vi "GaGeError.vi"(6 "Ingnore no sytem":bool=TRUE, 7 "source":string, 8 "error in (no error)":errorcluster, 9 "StopOnError (false)":bool, 10 "Error Code":i32, 11 "Handle Cluster":T1) -> (0 "error out":errorcluster, 3 "Error String":string)   [LabVIEW 2015]
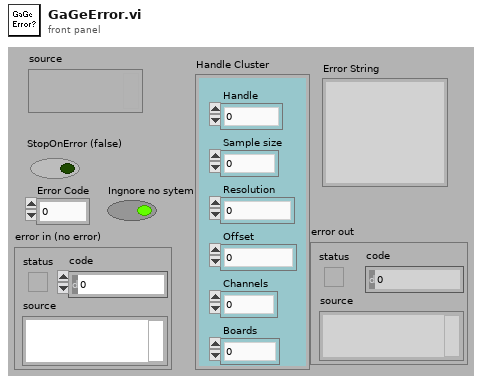
[diagram p1: front panel]
types:
  T1 = cluster{"Handle":u32, "Sample size":u32, "Resolution":i32, "Offset":i32, "Channels":u32, "Boards":u32}
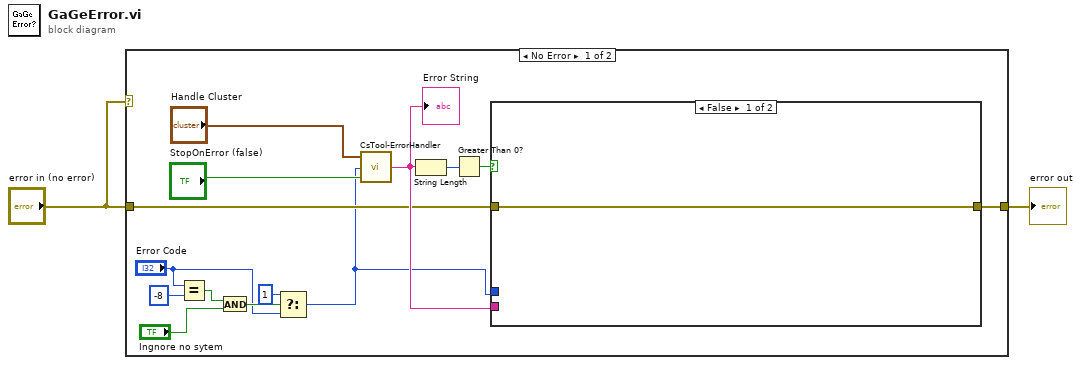
[diagram p0: block diagram]
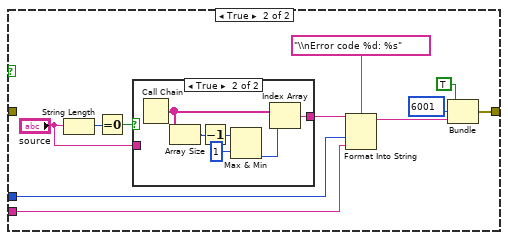
[diagram p2: hidden frame]
diagram:
  n1 = case shown="No Error" "error in (no error)" {
    tunnel: "error in (no error)" -> [w11 w36]
    tunnel: [w10 w36] -> w1
    frame No Error {
      n2 = Equal?(x="Error Code", y=-8) -> (x = y?=w8:bool)
      n3 = And(x=w8, y="Ingnore no sytem") -> (x .and. y?=w6:bool)
      n4 = Select(t=1, s=w6, f="Error Code") -> (s? t:f=w3:i32)
      n5 = call "CsTool-ErrorHandler.vi"("StopOnError (true)"="StopOnError (false)", "Error Code"=w3, "Handle Cluster"="Handle Cluster") -> ("Error String"=w12:string)
      "Error String" <- w12
      n6 = String Length(string=w12) -> (length=w14:i32)
      n7 = Greater Than 0?(x=w14) -> (x > 0?=w13:bool)
      n8 = case shown="False" w13 {
        tunnel: w3 -> [_ w20]
        tunnel: w12 -> [_ w19]
        tunnel: w11 -> [w17 _]
        tunnel: [w17 w18] -> w10
        frame False {
        }
        frame True {
          n9 = String Length(string="source") -> (length=w26:i32)
          n10 = Equal To 0?(x=w26) -> (x = 0?=w25:bool)
          n11 = case shown="True" w25 {
            tunnel: [w29 w33] -> w23
            tunnel: "source" -> [w29 _]
            frame False {
            }
            frame True {
              n12 = Call Chain() -> (call chain=w34:string[])
              n13 = Array Size(array=w34) -> (size(s)=w35:i32)
              n14 = Decrement(x=w35) -> (x-1=w32:i32)
              n15 = Max & Min(x=w32, y=1) -> (min(x,y)=w31:i32)  [unwired: 1 out]
              n16 = Index Array(array=w34, index=w31) -> (element=w33:string)
            }
          }
          n17 = Format Into String(format string="\\nError code %d: %s" ("Format String"), initial string=w23, w20, w19) -> (resulting string=w21:string)  [unwired: 1 in, 1 out]
          n18 = Bundle(TRUE, 6001, w21) -> (w18:errorcluster)  [unwired: 1 out]
        }
      }
    }
    frame Error {
    }
  }
  "error out" <- w1
